vi "Configure Trigger (Duration).vi"(0 "VISA resource name":refnum<visa-resource-name>, 1 "Duration Pattern Mask (0)":dbl, 2 "Limiting Condition (0: Greater Than)":i32(ring) items=["Greater Than", "Less Than", "Equal"], 5 "Trigger Source (0: Channel 1)":i32(ring) items=["Channel 1"=0, "Channel 2"=1, "EXT"=4, "AC Line"=6, "Digital 0"=7, "Digital 1"=8, "Digital 2"=9, "Digital 3"=10, "Digital 4"=11, "Digital 5"=12, "Digital 6"=13, "Digital 7"=14, "Digital 8"=15, "Digital 9"=16, "Digital 10"=17, "Digital 11"=18, "Digital 12"=19, "Digital 13"=20, "Digital 14"=21, "Digital 15"=22], 7 "Trigger Level (0)":dbl, 9 "Duration Pattern Value (0)":dbl, 11 "error in (no error)":errorcluster, 12 "Limiting Time (1E-6 s)":dbl=1e-06) -> (4 "VISA resource name out":refnum<visa-resource-name>, 15 "error out":errorcluster)   [LabVIEW 2023, in "RIGOL DS1054Z.lvlib"]
doc: "Configures duration trigger settings for an oscilloscope.\n\nNote:\nThis VI is only valid for DS1052D and DS1102D."
uses:
  RIGOL DS1054Z.lvlib
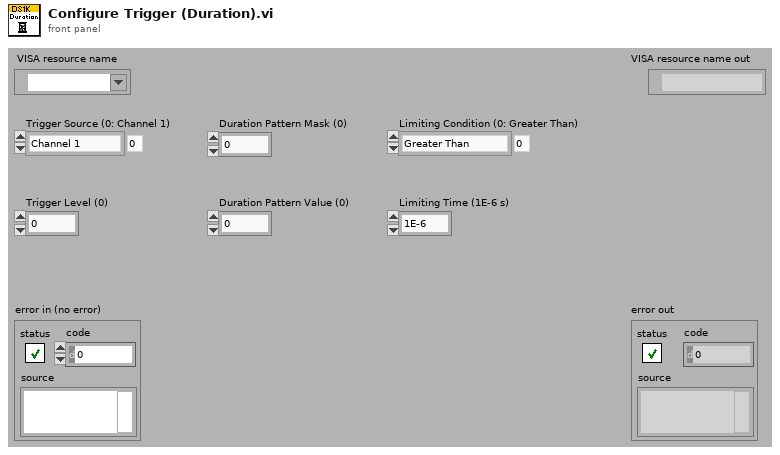
[diagram p1: front panel]
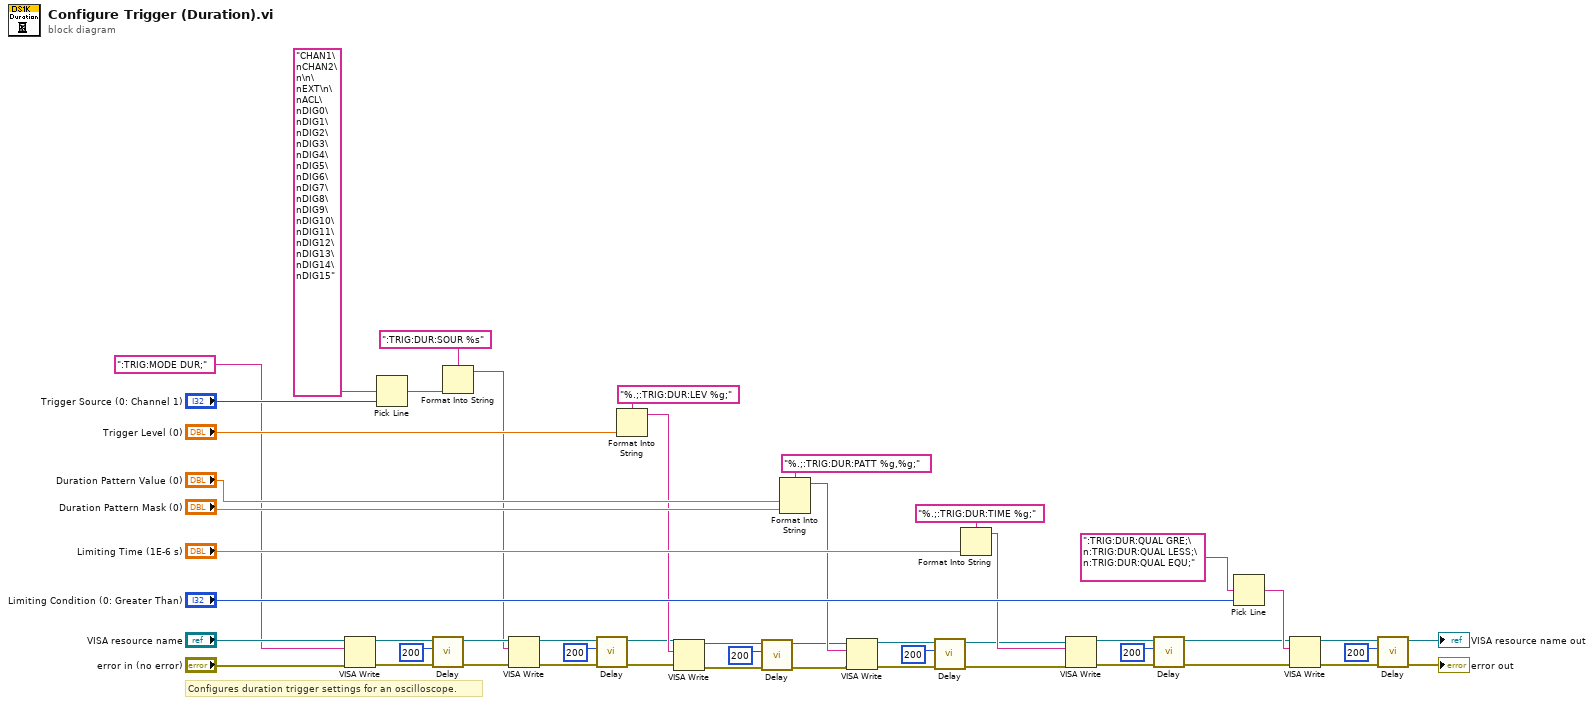
[diagram p0: block diagram]
diagram:
  # "Configures duration trigger settings for an oscilloscope."
  n1 = VISA Write(VISA resource name="VISA resource name", write buffer=":TRIG:MODE DUR;", error in (no error)="error in (no error)") -> (VISA resource name out=w10:refnum<visa-resource-name>, error out=w11:errorcluster)  [unwired: 1 out]
  n2 = Pick Line(multi-line string="CHAN1\nCHAN2\n\n\nEXT\n\nACL\nDIG0\nDIG1\nDIG2\nDIG3\nDIG4\nDIG5\nDIG6\nDIG7\nDIG8\nDIG9\nDIG10\nDIG11\nDIG12\nDIG13\nDIG14\nDIG15", line index="Trigger Source (0: Channel 1)") -> (output string=w3:string)  [unwired: 1 out]
  n3 = call "Delay.vi"("error in (no error)"=w11, "Delay (ms)"=u32 200, "VISA resource name"=w10) -> ("error out"=w7:errorcluster, "VISA resource name out"=w8:refnum<visa-resource-name>)  [unwired: 7 out]
  n4 = Format Into String(format string=":TRIG:DUR:SOUR %s", w3) -> (resulting string=w1:string)  [unwired: 2 in, 1 out]
  n5 = VISA Write(VISA resource name=w8, write buffer=w1, error in (no error)=w7) -> (VISA resource name out=w15:refnum<visa-resource-name>, error out=w14:errorcluster)  [unwired: 1 out]
  n6 = call "Delay.vi"("error in (no error)"=w14, "Delay (ms)"=u32 200, "VISA resource name"=w15) -> ("error out"=w12:errorcluster, "VISA resource name out"=w13:refnum<visa-resource-name>)  [unwired: 7 out]
  n7 = Format Into String(format string="%.;:TRIG:DUR:LEV %g;", "Trigger Level (0)") -> (resulting string=w17:string)  [unwired: 2 in, 1 out]
  n8 = VISA Write(VISA resource name=w13, write buffer=w17, error in (no error)=w12) -> (VISA resource name out=w33:refnum<visa-resource-name>, error out=w34:errorcluster)  [unwired: 1 out]
  n9 = call "Delay.vi"("error in (no error)"=w34, "Delay (ms)"=u32 200, "VISA resource name"=w33) -> ("error out"=w18:errorcluster, "VISA resource name out"=w19:refnum<visa-resource-name>)  [unwired: 7 out]
  n10 = Format Into String(format string="%.;:TRIG:DUR:PATT %g,%g;", "Duration Pattern Value (0)", "Duration Pattern Mask (0)") -> (resulting string=w20:string)  [unwired: 2 in, 1 out]
  n11 = VISA Write(VISA resource name=w19, write buffer=w20, error in (no error)=w18) -> (VISA resource name out=w24:refnum<visa-resource-name>, error out=w25:errorcluster)  [unwired: 1 out]
  n12 = call "Delay.vi"("error in (no error)"=w25, "Delay (ms)"=u32 200, "VISA resource name"=w24) -> ("error out"=w21:errorcluster, "VISA resource name out"=w22:refnum<visa-resource-name>)  [unwired: 7 out]
  n13 = Format Into String(format string="%.;:TRIG:DUR:TIME %g;", "Limiting Time (1E-6 s)") -> (resulting string=w26:string)  [unwired: 2 in, 1 out]
  n14 = VISA Write(VISA resource name=w22, write buffer=w26, error in (no error)=w21) -> (VISA resource name out=w30:refnum<visa-resource-name>, error out=w29:errorcluster)  [unwired: 1 out]
  n15 = call "Delay.vi"("error in (no error)"=w29, "Delay (ms)"=u32 200, "VISA resource name"=w30) -> ("error out"=w27:errorcluster, "VISA resource name out"=w28:refnum<visa-resource-name>)  [unwired: 7 out]
  n16 = Pick Line(multi-line string=":TRIG:DUR:QUAL GRE;\n:TRIG:DUR:QUAL LESS;\n:TRIG:DUR:QUAL EQU;", line index="Limiting Condition (0: Greater Than)") -> (output string=w40:string)  [unwired: 1 out]
  n17 = VISA Write(VISA resource name=w28, write buffer=w40, error in (no error)=w27) -> (VISA resource name out=w38:refnum<visa-resource-name>, error out=w36:errorcluster)  [unwired: 1 out]
  n18 = call "Delay.vi"("error in (no error)"=w36, "Delay (ms)"=u32 200, "VISA resource name"=w38) -> ("error out"=→"error out":errorcluster, "VISA resource name out"=→"VISA resource name out":refnum<visa-resource-name>)  [unwired: 7 out]
